vi "testKeithley.vi"() -> ()   [LabVIEW 2011, in "run.lvlib"]
uses:
  testing/run.lvlib
  Tools/DatabaseHelpers/DbConnection/DeviceDataBase/deviceDataBase.lvclass
  AnalogOutput.lvclass
panel:
  in  "physical channels":string="K2602a_Ao_00"
  in  "stop":bool
  in  "data":dbl[][][](array[numeric])=[[[0.0, 1.0], [1.0, 3.0], [1.5, 0.0]]]
  # "times s"
  # "voltage"
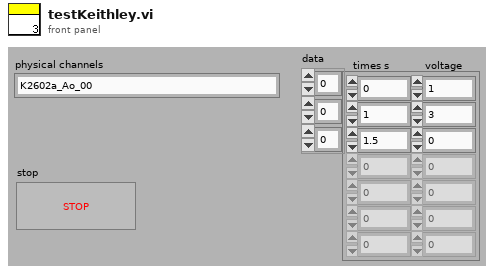
[diagram p1: front panel]
types:
  T1 = cluster{"Range":cluster{"current":dbl, "voltage":dbl}, "triggering_inUse":cluster{"start_trigger":string, "clock":string}, "Limits":cluster{"VoltageLimit":dbl, "CurrentLimit":dbl}}[]
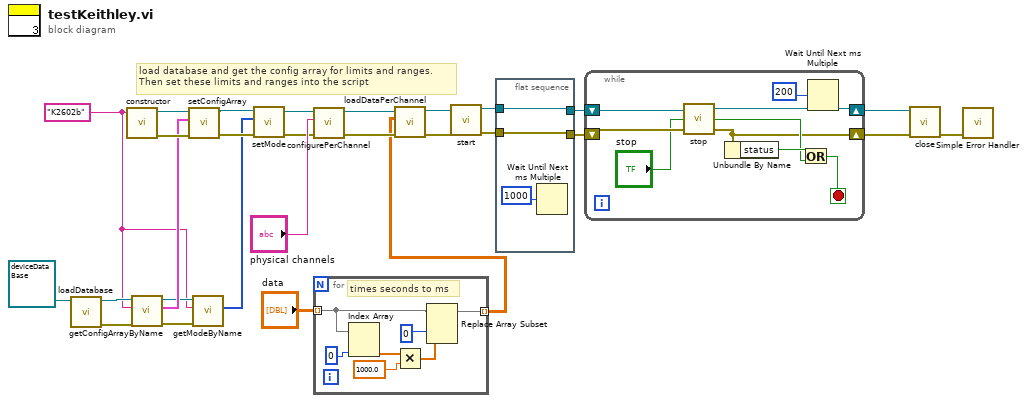
[diagram p0: block diagram]
diagram:
  w6 = "K2602b"
  # "load database and get the config array for limits and ranges.\nThen set these limits and ranges into the script"
  n1 = call "loadDatabase.vi"("deviceDataBase in"=refnum<class "deviceDataBase.lvclass"> refnum ("Tools.lvlib:DatabaseHelpers.lvlib:deviceDataBase.lvclass")) -> ("error out"=w16:errorcluster, "deviceDataBase out"=w17:refnum<class "deviceDataBase.lvclass">)  [unwired: 8 in, 1 out]
  n2 = call "constructor.vi"("deviceName"=w6) -> ("error out"=w21:errorcluster, "AnalogOutput out"=w22:refnum<class "AnalogOutput.lvclass">)  [unwired: 9 in]
  n3 = call "getConfigArrayByName.vi"("error in (no error)"=w16, "device_name"=w6, "deviceDataBase in"=w17) -> ("error out"=w7:errorcluster, "ConfigArray"=w15:T1, "deviceDataBase out"=w8:refnum<class "deviceDataBase.lvclass">)  [unwired: 6 in]
  n4 = call-dynamic "setConfigArray.vi"("error in (no error)"=w21, "ConfigArray"=w15, "AnalogOutput in"=w22) -> ("error out"=w4:errorcluster, "AnalogOutput out"=w5:refnum<class "AnalogOutput.lvclass">)  [unwired: 7 in]
  n5 = call "getModeByName.vi"("error in (no error)"=w7, "device_name"=w6, "deviceDataBase in"=w8) -> ("mode"=w1:enum16{"current", "voltage"}[])  [unwired: 6 in, 2 out]
  n6 = call "setMode.vi"("error in (no error)"=w4, "mode"=w1, "AnalogOutput in"=w5) -> ("error out"=w3:errorcluster, "AnalogOutput out"=w2:refnum<class "AnalogOutput.lvclass">)  [unwired: 7 in]
  n7 = call-dynamic "configurePerChannel.vi"("error in (no error)"=w3, "physical channels"="physical channels", "AnalogOutput in"=w2) -> ("error out"=w26:errorcluster, "AnalogOutput out"=w27:refnum<class "AnalogOutput.lvclass">)  [unwired: 7 in]
  n8 = for {
    tunnel: "data" -> [w31] mode=indexing
    tunnel: [w29] -> w9 mode=indexing
    # "times seconds to ms"
    n9 = Index Array(array=w31, index (col)=0) -> (element=w33:dbl[])  [unwired: 1 in]
    n10 = Multiply(x=w33, y=1000.0) -> (x*y=w30:dbl[])
    n11 = Replace Array Subset(array=w31, new element=w30, index (col)=0) -> (w29:dbl[][])  [unwired: 1 in]
  }
  n12 = call-dynamic "loadDataPerChannel.vi"("error in (no error)"=w26, "data"=w9, "AnalogOutput in"=w27) -> ("error out"=w19:errorcluster, "AnalogOutput out"=w20:refnum<class "AnalogOutput.lvclass">)  [unwired: 7 in]
  n13 = call-dynamic "start.vi"("error in (no error)"=w19, "AnalogOutput in"=w20) -> ("error out"=w11:errorcluster, "AnalogOutput out"=w13:refnum<class "AnalogOutput.lvclass">)  [unwired: 8 in]
  n14 = flat-sequence {
    tunnel: [w38] -> w14
    tunnel: w13 -> [w38]
    tunnel: [w37] -> w12
    tunnel: w11 -> [w37]
    frame #0 {
      n15 = Wait Until Next ms Multiple(millisecond multiple=1000) -> ()  [unwired: 1 out]
    }
  }
  n16 = while {
    shift-right: [w46] -> w25
    shift-left: w14 -> [w47]
    shift-right: [w40] -> w24
    shift-left: w12 -> [w45]
    stop <- w41 stop-if-true
    n17 = call-dynamic "stop.vi"("error in (no error)"=w45, "stop"="stop", "AnalogOutput in"=w47) -> ("error out"=w40:errorcluster, "Stopped"=w42:bool, "AnalogOutput out"=w46:refnum<class "AnalogOutput.lvclass">)
    n18 = Unbundle By Name(w40) -> ("status"=w43:bool)
    n19 = Or(x=w43, y=w42) -> (x .or. y?=w41:bool)
    n20 = Wait Until Next ms Multiple(millisecond multiple=200) -> ()  [unwired: 1 out]
  }
  n21 = call-dynamic "close.vi"("error in (no error)"=w24, "AnalogOutput in"=w25) -> ("error out"=w23:errorcluster)  [unwired: 9 in]
  n22 = call <vilib>:"Simple Error Handler.vi"("error in (no error)"=w23) -> ()  [unwired: 4 in, 5 out]
